vi "Synchronize Control Panel.vi"(8 "error in (no error)":errorcluster, 11 "LakeShore 335 in":refnum<class "LakeShore 335.lvclass">) -> (0 "error out":errorcluster, 3 "LakeShore 335 out":refnum<class "LakeShore 335.lvclass">)   [LabVIEW 2015, in "LakeShore 335.lvclass"]
uses:
  LakeShore 335.lvclass
  LakeShore335 Front Panel Data.ctl
  LakeShore335 Heater Ranges.ctl
  Neocera/Neocera Set Point Aproach.ctl
  Instrument/Read VISA Resource.vi
  Instrument/Write VISA Resource.vi
  OO Devices/Device/Device.lvclass
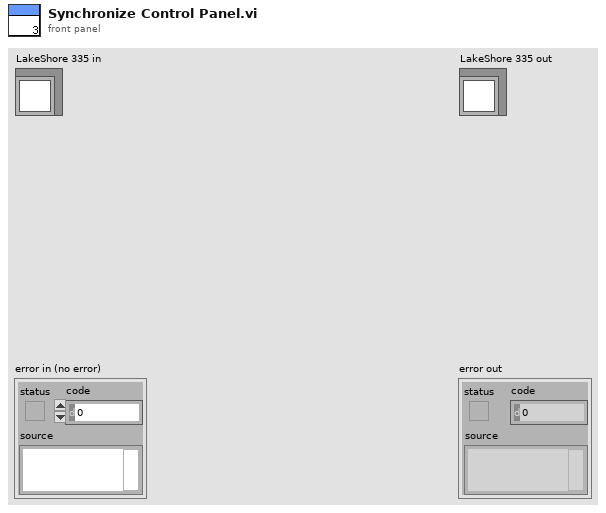
[diagram p1: front panel]
types:
  T1 = typedef "LakeShore335 Front Panel Data.ctl" = cluster{"Heater":bool, "A":bool, "B":bool, " RAW":bool, "Set point":dbl, "Set Heater Range":T2, "Approach":T3, "Ramp rate, K/min":dbl}
  T2 = typedef "LakeShore335 Heater Ranges.ctl" = enum16{"0 (Off)", "1 Low", "2 Medium", "3 High"}
  T3 = typedef "Neocera Set Point Aproach.ctl" = enum16{"Instant", "Ramp"}
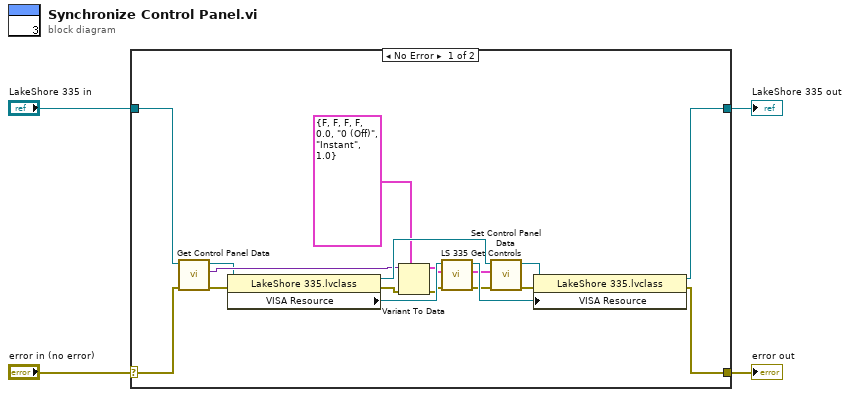
[diagram p0: block diagram]
diagram:
  n1 = case shown="No Error" "error in (no error)" {
    selector: "error in (no error)" -> [w5 w24]
    tunnel: [w6 w24] -> w3
    tunnel: [w7 w23] -> w1
    tunnel: "LakeShore 335 in" -> [w8 w23]
    frame No Error {
      n2 = call-dynamic "Get Control Panel Data.vi"("error in (no error)"=w5, "Device in"=w8) -> ("error out"=w16:errorcluster, "Data"=w13:variant, "Device out"=w9:refnum<class "LakeShore 335.lvclass">)  [unwired: 7 in]
      n3 = property class="LakeShore 335.lvclass"(reference=w9, error in=w16) -> (reference out=w18:refnum<class "LakeShore 335.lvclass">, error out=w17:errorcluster, "VISA Resource"=w22:refnum<visa-resource-name>)
      n4 = Variant To Data(error in=w17, type=T1 {"Heater"=FALSE, "A"=FALSE, "B"=FALSE, " RAW"=FALSE, "Set point"=0.0, "Set Heater Range"=enum."0 (Off)", "Approach"=enum."Instant", "Ramp rate, K/min"=1.0} ("Data"), Variant=w13) -> (data=w12:T1, error out=w11:errorcluster)
      n5 = call "LS 335 Get Controls.vi"("error in (no error)"=w11, "Control Panel Data"=w12, "VISA resource name"=w22) -> ("error out"=w14:errorcluster, "Control Panel Data Out"=w15:T1, "VISA Resource Name Out"=w21:refnum<visa-resource-name>)  [unwired: 6 in]
      n6 = call "Set Control Panel Data.vi"("error in (no error)"=w14, "Data"=w15, "Device in"=w18) -> ("error out"=w20:errorcluster, "Device out"=w19:refnum<class "LakeShore 335.lvclass">)  [unwired: 7 in]
      n7 = property class="LakeShore 335.lvclass"(reference=w19, error in=w20, "VISA Resource"=w21) -> (reference out=w7:refnum<class "LakeShore 335.lvclass">, error out=w6:errorcluster)
    }
    frame Error {
    }
  }
  "error out" <- w3
  "LakeShore 335 out" <- w1
